vi "target1.vi"() -> ()   [LabVIEW 2023]
panel:
  out "x+y":dbl
  in  "y":dbl
  out "x+1":dbl
  in  "x":dbl
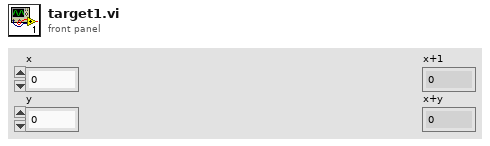
[diagram p1: front panel]
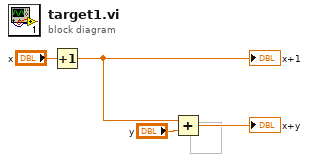
[diagram p0: block diagram]
diagram:
  n1 = Increment(x="x") -> (x+1=w3:dbl)
  "x+1" <- w3
  n2 = Add(x=w3, y="y") -> (x+y=→"x+y":dbl)
